vi "SQL-LV Generate Insert Method.vi"(8 "error in (no error)":errorcluster, 9 "SQL-LV Control Paths":T1, 10 "Table Name":string, 11 "Save as":path) -> (0 "error out":errorcluster, 3 "Save as out":path)   [LabVIEW 2021]
uses:
  SQL-LV Table Control Paths.ctl
  edt.lib/vi_script.lib/Control Replacement Param.ctl
  DB Method Enum.ctl
  edt.lib/vi_script.lib/Constant Replacement Param.ctl
  edt.lib/vi_script.lib/Replace Control in VI (Scalar).vi
  edt.lib/vi_script.lib/Replace Constant in VI (Scalar).vi
  edt.lib/vi_script.lib/EDT VI Script.lvlib
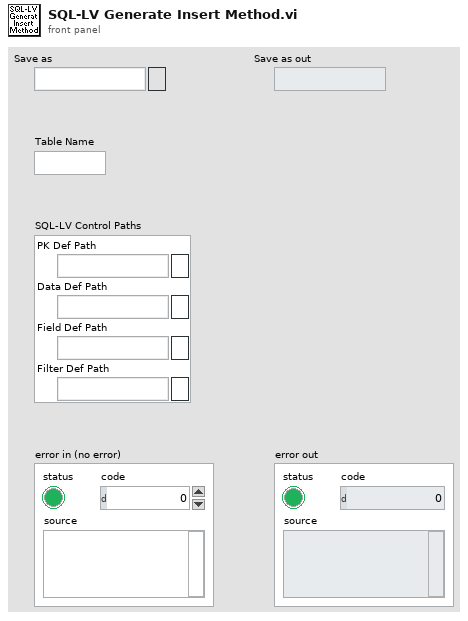
[diagram p1: front panel]
types:
  T1 = typedef "SQL-LV Table Control Paths.ctl" = cluster{"PK Def Path":path, "Data Def Path":path, "Field Def Path":path, "Filter Def Path":path}
  T2 = typedef "EDT VI Script.lvlib/Constant Replacement Param.ctl" = cluster{"Label.Text":string, "Value":variant}
  T3 = typedef "DB Method Enum.ctl" = enum16{"Insert", "Delete", "Select", "Update", "List"}
  T4 = typedef "EDT VI Script.lvlib/Control Replacement Param.ctl" = cluster{"Placeholder Name":string, "CTL File Path":path, "Indicator":bool}
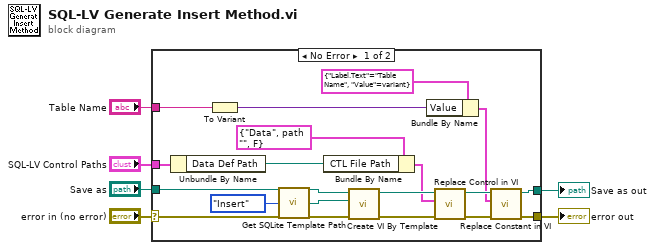
[diagram p0: block diagram]
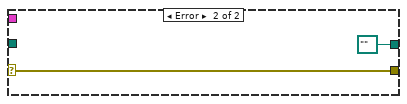
[diagram p2: hidden frame]
diagram:
  n1 = case shown="No Error" "error in (no error)" {
    selector: "error in (no error)" -> [w21 w25]
    tunnel: [w10 path "" ("Save as out")] -> w6
    tunnel: "Save as" -> [w8 _]
    tunnel: [w11 w25] -> w4
    tunnel: "SQL-LV Control Paths" -> [w18 _]
    tunnel: "Table Name" -> [w14 _]
    frame No Error {
      n2 = Unbundle By Name(w18) -> ("Data Def Path"=w17:path)
      n3 = To Variant(anything=w14) -> (Variant=w13:variant)
      n4 = call "Get SQLite Template Path.vi"("Template Type"=DB_Method_Enum."Insert") -> ("Template Path"=w7:path)
      n5 = Bundle By Name(cluster=T4 {"Placeholder Name"="Data", "CTL File Path"=path "", "Indicator"=FALSE} ("Control Replacement Param"), "CTL File Path"=w17) -> (w9:T4)
      n6 = call "Create VI By Template.vi"("error in"=w21, "Template VI Path"=w7, "Save as"=w8) -> ("error out"=w19:errorcluster, "Save as out"=w20:path)  [unwired: 7 in]
      n7 = Bundle By Name(cluster=T2 {"Label.Text"="Table Name", "Value"=variant} ("Constant Replacement Params"), "Value"=w13) -> (w12:T2)
      n8 = call-poly "Replace Control in VI.vi"("error in"=w19, "Control Replacement Params"=w9, "Original VI"=w20) -> ("error out"=w16:errorcluster, "Save as out"=w23:path)  [unwired: 7 in]
      n9 = call-poly "Replace Constant in VI.vi"("error in"=w16, "Constant Replacement Params"=w12, "Original VI"=w23) -> ("error out"=w11:errorcluster, "Save as out"=w10:path)  [unwired: 7 in]
    }
    frame Error {
    }
  }
  "Save as out" <- w6
  "error out" <- w4
